vi "Read Pattern Name.vi"(8 "error in (no error)":errorcluster, 11 "SPI Root Pattern Creator in":refnum<class "SPI Root Pattern Creator.lvclass">) -> (0 "error out":errorcluster, 2 "Pattern Name":string, 3 "SPI Root Pattern Creator out":refnum<class "SPI Root Pattern Creator.lvclass">)   [LabVIEW 2018, in "SPI Root Pattern Creator.lvlib" / "SPI Root Pattern Creator.lvclass"]
uses:
  SPI Root Pattern Creator.lvclass
  SPI Root Pattern Creator.lvclass/SPI Root Pattern Creator.ctl
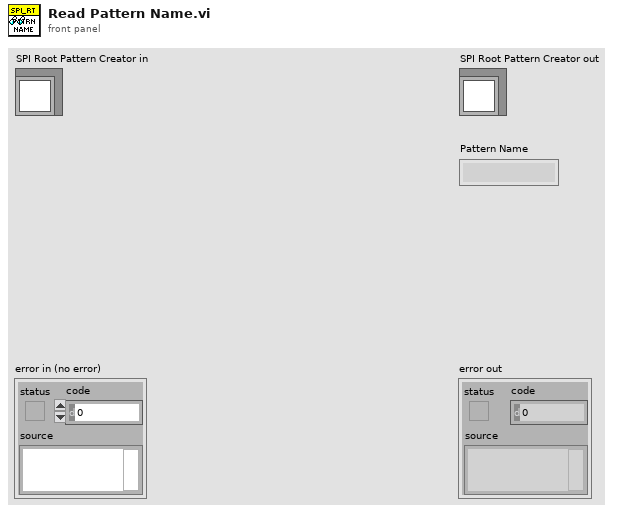
[diagram p1: front panel]
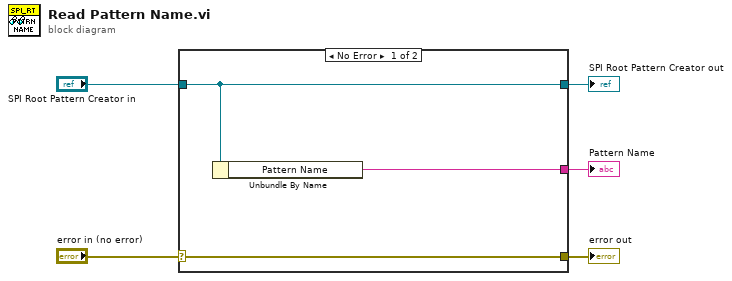
[diagram p0: block diagram]
diagram:
  n1 = case shown="No Error" "error in (no error)" {
    selector: "error in (no error)" -> [w8 w9]
    tunnel: [w8 w9] -> w4
    tunnel: [w7 w10] -> w2
    tunnel: "SPI Root Pattern Creator in" -> [w7 w10]
    tunnel: [w6 _] -> w1
    frame No Error {
      n2 = Unbundle By Name(w7) -> ("Pattern Name"=w6:string)
    }
    frame Error {
    }
  }
  "error out" <- w4
  "SPI Root Pattern Creator out" <- w2
  "Pattern Name" <- w1
